vi "trio_position.vi"(8 "error in":errorcluster, 10 "Axis":i16, 11 "Trio handle":refnum<k7>) -> (0 "error out":errorcluster, 2 "Position":dbl, 3 "Handle out":refnum<k7>)   [LabVIEW 2017]
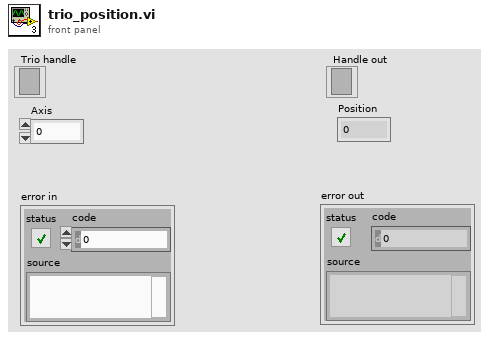
[diagram p1: front panel]
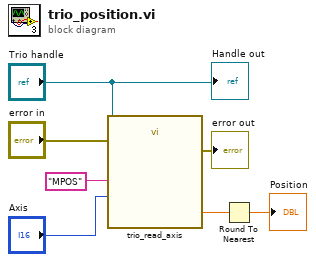
[diagram p0: block diagram]
diagram:
  n1 = call "trio_read_axis.vi"("Axis"="Axis", "error in (no error)"="error in", "Variable"="MPOS", "reference in"="Trio handle") -> ("error out"=→"error out":errorcluster, "Value"=w1:dbl)  [unwired: 5 in, 1 out]
  n2 = Round To Nearest(number=w1) -> (nearest integer value=→"Position":dbl)
  "Handle out" <- "Trio handle"
